vi "SetHe4Pressure.vi"() -> ()   [LabVIEW 2021, in "Mercury iXX.lvlib"]
uses:
  <instrlib>/Mercury iXX/Mercury iXX.lvlib
  <instrlib>/Mercury iXX/Public/Libraries/Pressure/Controls/Pressure Device (Read).ctl
  <instrlib>/Mercury iXX/Public/Controls/Manufacturing Data.ctl
  <instrlib>/Mercury iXX/Public/Libraries/Pressure/Controls/Pressure Sensor Type.ctl
  <instrlib>/Mercury iXX/Public/Libraries/Pressure/Controls/Calibration Cluster.ctl
  <instrlib>/Mercury iXX/Public/Libraries/Pressure/Controls/Calibration Interpolation.ctl
  <instrlib>/Mercury iXX/Public/Libraries/Pressure/Controls/Loop Cluster.ctl
  <instrlib>/Mercury iXX/Public/Libraries/Pressure/Controls/Pressure Signals Cluster.ctl
  <instrlib>/Mercury iXX/Public/Controls/Comms Transport Layer.ctl
  <instrlib>/Mercury iXX/Public/Controls/ISOBus Address.ctl
  <instrlib>/Mercury iXX/Private/Controls/Lookup Reference FGV Enum.ctl
  <instrlib>/Mercury iXX/Public/Libraries/System/Open/Open System.vi
  <instrlib>/Mercury iXX/Public/Libraries/System/Read/Catalogue (Read).vi
  <instrlib>/Mercury iXX/Public/Libraries/System/Open/Open Device.vi
  <instrlib>/Mercury iXX/Public/Libraries/Pressure/Configuration/Set/Pressure Device (Set).vi
  <instrlib>/Mercury iXX/Public/Libraries/Pressure/Configuration/Read/Pressure Device (Read).vi
  <instrlib>/Mercury iXX/Public/Libraries/System/Set/Date (Set).vi
  <instrlib>/Mercury iXX/Public/Libraries/System/Read/DateTime (Read).vi
  <instrlib>/Mercury iXX/Public/Libraries/System.lvlib
  <instrlib>/Mercury iXX/Public/Libraries/System/Set/Time (Set).vi
  <instrlib>/Mercury iXX/Public/Libraries/Pressure.lvlib
panel:
  out "Device Details":T1
  out "time stamp":timestamp
  out "Devices":string[](array[string])
  out "Set Date Response":string
  out "Set Time Response":string
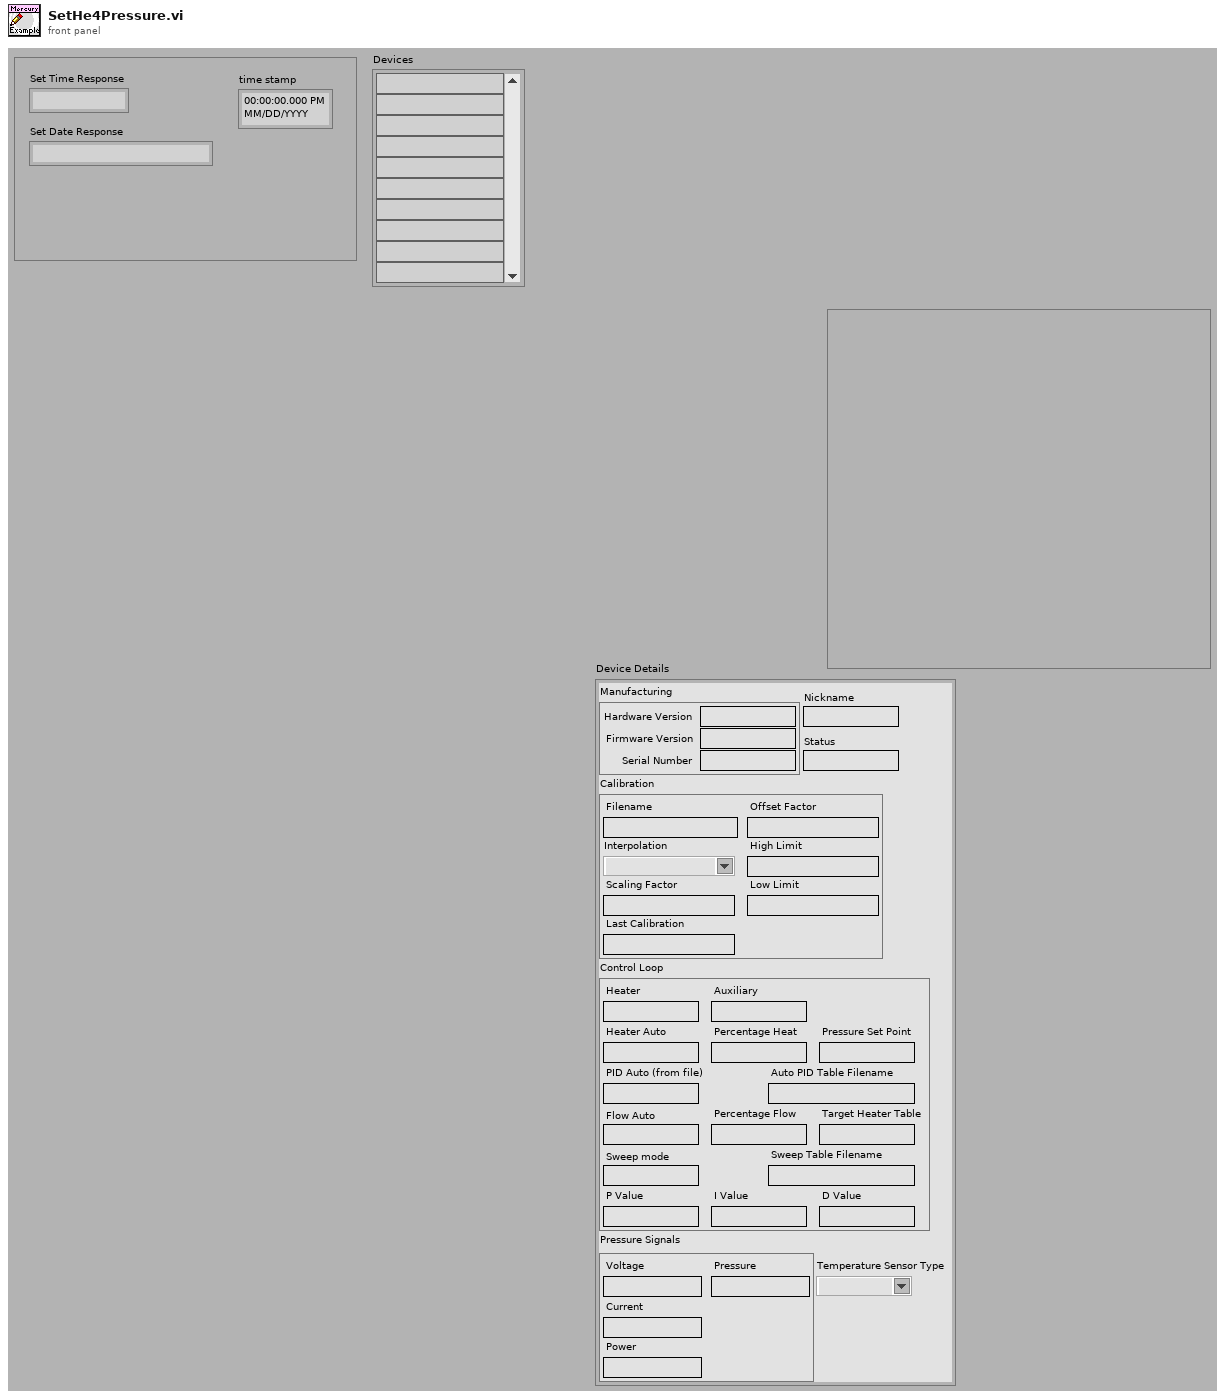
[diagram p1: front panel]
types:
  T1 = typedef "Mercury iXX.lvlib/Pressure.lvlib/Pressure Device (Read).ctl" = cluster{"Manufacturing":T2, "Temperature Sensor Type":T3, "Calibration":T4, "Control Loop":T6, "Pressure Signals":T7, "Nickname":string, "Status":string}
  T2 = typedef "Mercury iXX.lvlib/Manufacturing Data.ctl" = cluster{"Hardware Version":string, "Firmware Version":string, "Serial Number":string}
  T3 = typedef "Mercury iXX.lvlib/Pressure.lvlib/Pressure Sensor Type.ctl" = string
  T4 = typedef "Mercury iXX.lvlib/Pressure.lvlib/Calibration Cluster.ctl" = cluster{"Filename":string, "Interpolation":T5, "Scaling Factor":string, "Offset Factor":string, "High Limit":string, "Low Limit":string, "Last Calibration":string}
  T5 = typedef "Mercury iXX.lvlib/Pressure.lvlib/Calibration Interpolation.ctl" = string
  T6 = typedef "Mercury iXX.lvlib/Pressure.lvlib/Loop Cluster.ctl" = cluster{"Heater":string, "Auxiliary":string, "Heater Auto":string, "Percentage Heat":string, "Pressure Set Point":string, "PID Auto (from file)":string, "P Value":string, "I Value":string, "D Value":string, "Auto PID Table Filename":string, "Flow Auto":string, "Target Heater Table":string, "Sweep mode":string, "Sweep Table Filename":string, "Percentage Flow":string}
  T7 = typedef "Mercury iXX.lvlib/Pressure.lvlib/Pressure Signals Cluster.ctl" = cluster{"Voltage":string, "Current":string, "Power":string, "Pressure":string}
  T8 = typedef "Mercury iXX.lvlib/ISOBus Address.ctl" = i32
  T9 = typedef "Mercury iXX.lvlib/Comms Transport Layer.ctl" = enum16{"Ethernet TCP/IP", "USB", "ISOBus - RS-232", "GPIB"}
  T10 = typedef "Mercury iXX.lvlib/Mercury Reference.ctl" = cluster{"Comms":refnum<visa-resource-name>, "Device ID":string[], "Comms Layer":T9, "Command":string, "Query reference":T11}
  T11 = typedef "Mercury iXX.lvlib/Query Dynamic Reference.ctl" = refnum<vi>
  T12 = typedef "Mercury iXX.lvlib/Response String.ctl" = string
  T13 = typedef "Mercury iXX.lvlib/Lookup Reference FGV Enum.ctl" = enum16{"Check VISA", "Get VI Ref", "Set VI ref", "Delete Single Ref", "Clear All"}
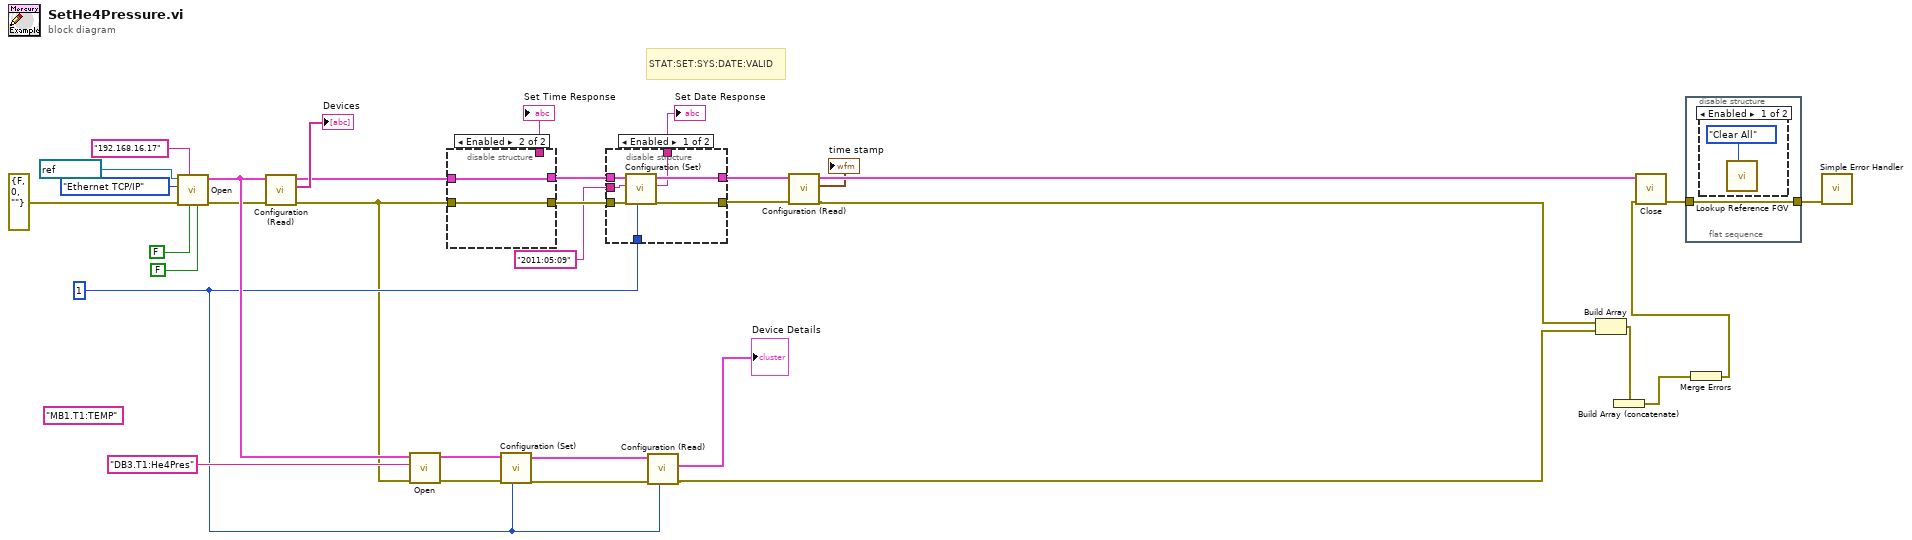
[diagram p0: block diagram]
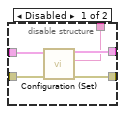
[diagram p4: hidden frame]
diagram:
  (unwired) "MB1.T1:TEMP" ("Device Identifier")
  w12 = T8 1 ("ISOBUS address")
  # "STAT:SET:SYS:DATE:VALID"
  n1 = call-poly <instrlib>:"Open.vi"("Clear Previous Connections (False)"=FALSE ("Reset (True)"), "ID Query (True)"=FALSE, "IP Address"="192.168.16.17", "error in (no error)"=errorcluster {"status"=FALSE, "code"=0, "source"=""}, "Comms Layer"=Comms_Transport_Layer."Ethernet TCP/IP", "VISA resource name"=refnum<visa-resource-name> "COM1") -> ("error out"=w20:errorcluster, "Mercury Reference Out"=w21:T10)  [unwired: 1 in, 3 out]
  n2 = call-poly <instrlib>:"Configuration (Read).vi"("error in"=w20, "Mercury Reference In"=w21) -> ("error out"=w6:errorcluster, "Devices"=→"Devices":string[], "Mercury Reference Out"=w18:T10)  [unwired: 1 in, 6 out]
  n3 = call-poly <instrlib>:"Open.vi"("error in (no error)"=w6, "Device Identifier"="DB3.T1:He4Pres", "Mercury Reference In"=w21) -> ("error out"=w17:errorcluster, "Mercury Reference Out"=w16:T10)  [unwired: 1 in, 6 out]
  n4 = disable-structure shown="Enabled" {
    disable-tunnel: w18 -> [w39 w41]
    disable-tunnel: w6 -> [w38 w40]
    disable-tunnel: [w37 w40] -> w31
    disable-tunnel: [w36 w41] -> w30
    disable-tunnel: [w35 _] -> w29
    frame Disabled {
      n5 = call-poly <instrlib>:"Configuration (Set).vi"("error in"=w38, "Mercury Reference In"=w39) -> ("error out"=w37:errorcluster, "Response"=w35:T12, "Mercury Reference Out"=w36:T10)  [unwired: 6 in, 1 out]
    }
    frame Enabled {
    }
  }
  "Set Time Response" <- w29
  n6 = call-poly <instrlib>:"Configuration (Set).vi"("ISOBUS address"=w12, "error in"=w17, "Mercury Reference In"=w16) -> ("error out"=w14:errorcluster, "Mercury Reference Out"=w13:T10)  [unwired: 1 in, 6 out]
  n7 = disable-structure shown="Enabled" {
    disable-tunnel: w31 -> [w48 w49]
    disable-tunnel: w30 -> [w47 w50]
    disable-tunnel: [w46 w50] -> w9
    disable-tunnel: [w45 w49] -> w8
    disable-tunnel: [w44 _] -> w28
    disable-tunnel: "2011:05:09" ("Date") -> [w43 _]
    disable-tunnel: w12 -> [w42 _]
    frame Enabled {
      n8 = call-poly <instrlib>:"Configuration (Set).vi"("ISOBUS address"=w42, "error in"=w48, "Date"=w43, "Mercury Reference In"=w47) -> ("error out"=w45:errorcluster, "Response"=w44:T12, "Mercury Reference Out"=w46:T10)  [unwired: 5 out]
    }
    frame Disabled {
    }
  }
  "Set Date Response" <- w28
  n9 = call-poly <instrlib>:"Configuration (Read).vi"("ISOBUS address"=w12, "error in"=w14, "Mercury Reference In"=w13) -> ("error out"=w15:errorcluster, "Device Details"=→"Device Details":T1)  [unwired: 7 out]
  n10 = call-poly <instrlib>:"Configuration (Read).vi"("error in"=w8, "Mercury Reference In"=w9) -> ("error out"=w10:errorcluster, "time stamp"=→"time stamp":timestamp, "Mercury Reference Out"=w11:T10)  [unwired: 1 in, 6 out]
  n11 = Build Array(w10, w15) -> (w3:errorcluster[])
  n12 = Build Array (concatenate)(w3) -> (w2:errorcluster[])
  n13 = flat-sequence {
    tunnel: [w51] -> w23
    tunnel: w22 -> [w51]
    frame #0 {
      n14 = disable-structure shown="Enabled" {
        frame Enabled {
          n15 = call <instrlib>:"Lookup Reference FGV.vi"("State"=Lookup_Reference_FGV_Enum."Clear All") -> ()  [unwired: 4 in, 7 out]
        }
        frame Disabled {
        }
      }
    }
  }
  n16 = Merge Errors(w2) -> (w24:errorcluster)
  n17 = call <instrlib>:"Close.vi"("error in (no error)"=w24, "Mercury Reference"=w11) -> ("error out"=w22:errorcluster)  [unwired: 9 out]
  n18 = call <vilib>:"Simple Error Handler.vi"("error in (no error)"=w23) -> ()  [unwired: 1 in, 8 out]
